vi "ISX3_Cmd_CalibrationACK.vi"(1 "ACK / NACK":bool) -> (0 "ACK / NACK Calibration cmd":u8[](array[numeric]))   [LabVIEW 2012, in "Sciospec ISX3 Impedance Analyzer.lvlib"]
uses:
  Sciospec ISX3 Impedance Analyzer.lvlib
panel:
  # "This VI generates the command for a Calibration Acknowledge (CACK) or Calibration Not Acknowledge (CNACK).\nThis command must be send to answer the calibration interaction request for open and short."
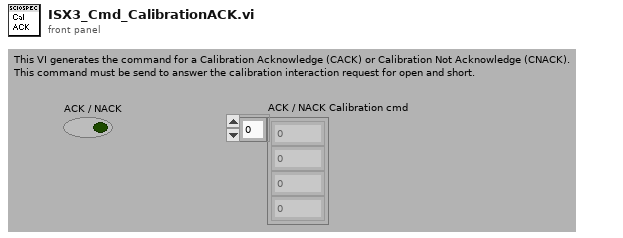
[diagram p1: front panel]
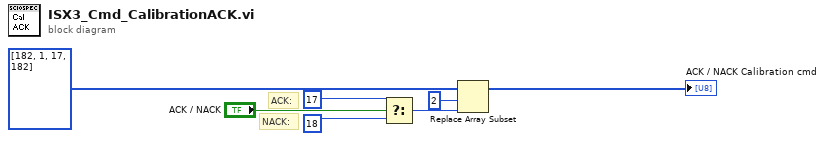
[diagram p0: block diagram]
diagram:
  # "NACK:"
  # "ACK:"
  n1 = Select(t=u8 17, s="ACK / NACK", f=u8 18) -> (s? t:f=w4:u8)
  n2 = Replace Array Subset(array=u8[] [182, 1, 17, 182], new element=w4, index=2 ("Index")) -> (→"ACK / NACK Calibration cmd":u8[])
